vi "SmartMotor_single motor update params and go.vi"(0 "VISA In":refnum<visa-resource-name>, 5 "Commands":string[](array[string]), 7 "MotorSpecifier(None)":T1, 9 "SendGo? (T)":bool=TRUE, 11 "error in":errorcluster, 12 "InterParamWait (5ms)":u32=5, 13 "ReadWait":u32=50, 14 "Semaphore Timeout (5000)":i32=5000) -> (4 "VISA out":refnum<visa-resource-name>, 6 "Cmd Str out":string, 15 "error out":errorcluster)   [LabVIEW 2020]
doc: "Developed by: Kevin Thompson\nThompson Engineering\nkevin@thompsonengineering.net\n(510) 673-3614"
uses:
  TD SerialBusMotorSpecifier_enum.ctl
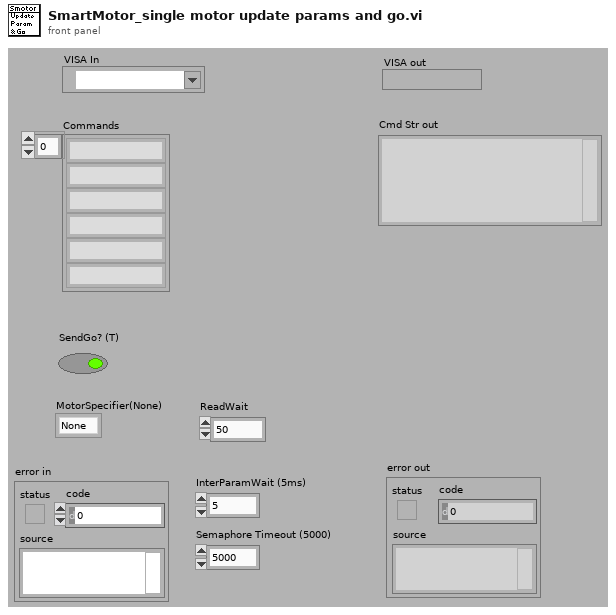
[diagram p1: front panel]
types:
  T1 = typedef "TD SerialBusMotorSpecifier_enum.ctl" = enum16{"None", "Global", "M1", "M2", "M3"}
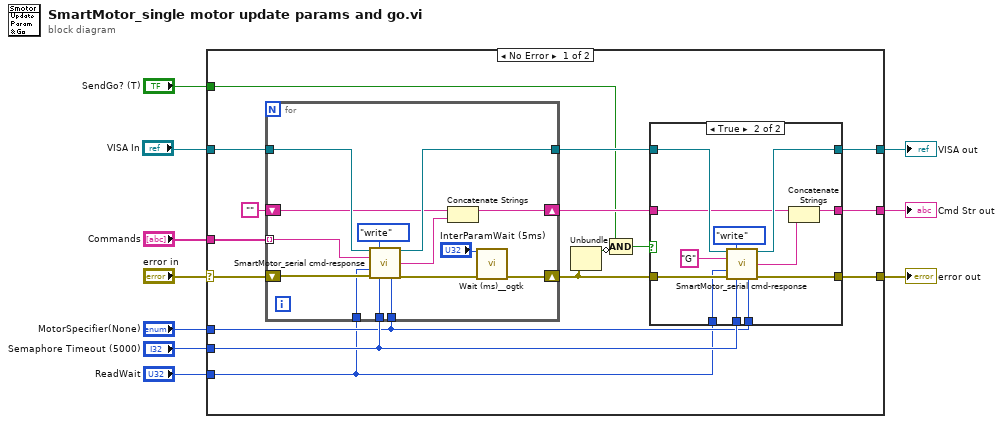
[diagram p0: block diagram]
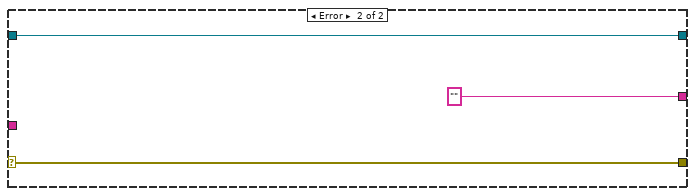
[diagram p3: hidden frame]
diagram:
  n1 = case shown="No Error" "error in" {
    selector: "error in" -> [w13 w57]
    tunnel: [w26 w57] -> w10
    tunnel: [w21 w58] -> w9
    tunnel: "VISA In" -> [w20 w58]
    tunnel: [w17 ""] -> w6
    tunnel: "Semaphore Timeout (5000)" -> [w16 _]
    tunnel: "SendGo? (T)" -> [w15 _]
    tunnel: "MotorSpecifier(None)" -> [w14 _]
    tunnel: "Commands" -> [w12 _]
    tunnel: "ReadWait" -> [w11 _]
    frame No Error {
      n2 = for {
        shift-right: [w55] -> w25
        shift-left: w13 -> [w54]
        tunnel: w20 -> [w53]
        tunnel: [w52] -> w22
        tunnel: w16 -> [w51]
        shift-right: [w49] -> w18
        shift-left: "" -> [w50]
        tunnel: w14 -> [w48]
        tunnel: w12 -> [w47] mode=indexing
        tunnel: w11 -> [w42]
        n3 = call "SmartMotor_serial cmd-response.vi"("VISA In"=w53, "mode"=enum16{"wr & rd", "write", "read"}."write", "cmd"=w47, "ReadWait"=w42, "error in"=w54, "Sem Timeout (5000)"=w51, "MotorSpecifier(None)"=w48) -> ("VISA out"=w52:refnum<visa-resource-name>, "cmd str out"=w43:string, "error out"=w45:errorcluster)  [unwired: 4 in, 2 out]
        n4 = Concatenate Strings(w50, w43) -> (w49:string)
        n5 = call <userlib>:"Wait (ms)__ogtk.vi"("error in (no error)"=w45, "milliseconds to wait"="InterParamWait (5ms)") -> ("error out"=w55:errorcluster)  [unwired: 8 in, 1 out]
      }
      n6 = Unbundle(w25) -> ("status"=w24:bool)  [unwired: 2 out]
      n7 = Compound Arithmetic op=AND(w15, invert w24) -> (w23:bool)
      n8 = case shown="True" w23 {
        tunnel: w25 -> [w29 w40]
        tunnel: [w29 w39] -> w26
        tunnel: w22 -> [w28 w37]
        tunnel: [w28 w36] -> w21
        tunnel: w16 -> [_ w35]
        tunnel: w18 -> [w27 w34]
        tunnel: [w27 w32] -> w17
        tunnel: w14 -> [_ w31]
        tunnel: w11 -> [_ w30]
        frame False {
        }
        frame True {
          n9 = call "SmartMotor_serial cmd-response.vi"("VISA In"=w37, "mode"=enum16{"wr & rd", "write", "read"}."write", "cmd"="G" ("String to Write"), "ReadWait"=w30, "error in"=w40, "Sem Timeout (5000)"=w35, "MotorSpecifier(None)"=w31) -> ("VISA out"=w36:refnum<visa-resource-name>, "cmd str out"=w33:string, "error out"=w39:errorcluster)  [unwired: 4 in, 2 out]
          n10 = Concatenate Strings(w34, w33) -> (w32:string)
        }
      }
    }
    frame Error {
    }
  }
  "error out" <- w10
  "VISA out" <- w9
  "Cmd Str out" <- w6
